vi "Periodic Tasks.vi"(8 "error in":errorcluster) -> ()   [LabVIEW 2023]
doc: "This VI runs in parallel to other tasks. It can contain as many user-defined periodic loops as you need. These can carry out PID or other sorts of timed response."
uses:
  <vilib>/Rock Robotics/WPI/DriverStation/WPI_DriverStationAllianceInfo.ctl
  <vilib>/Rock Robotics/Network Tables/NT Read String.vi
  <vilib>/Rock Robotics/Network Tables/NT Write String.vi
  GeneralPurpose/AllianceColorGlobal.vi
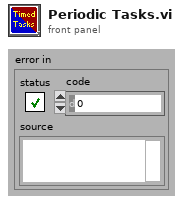
[diagram p1: front panel]
types:
  T1 = typedef "WPI_DriverStationAllianceInfo.ctl" = enum16{"Red", "Blue", "Invalid"}
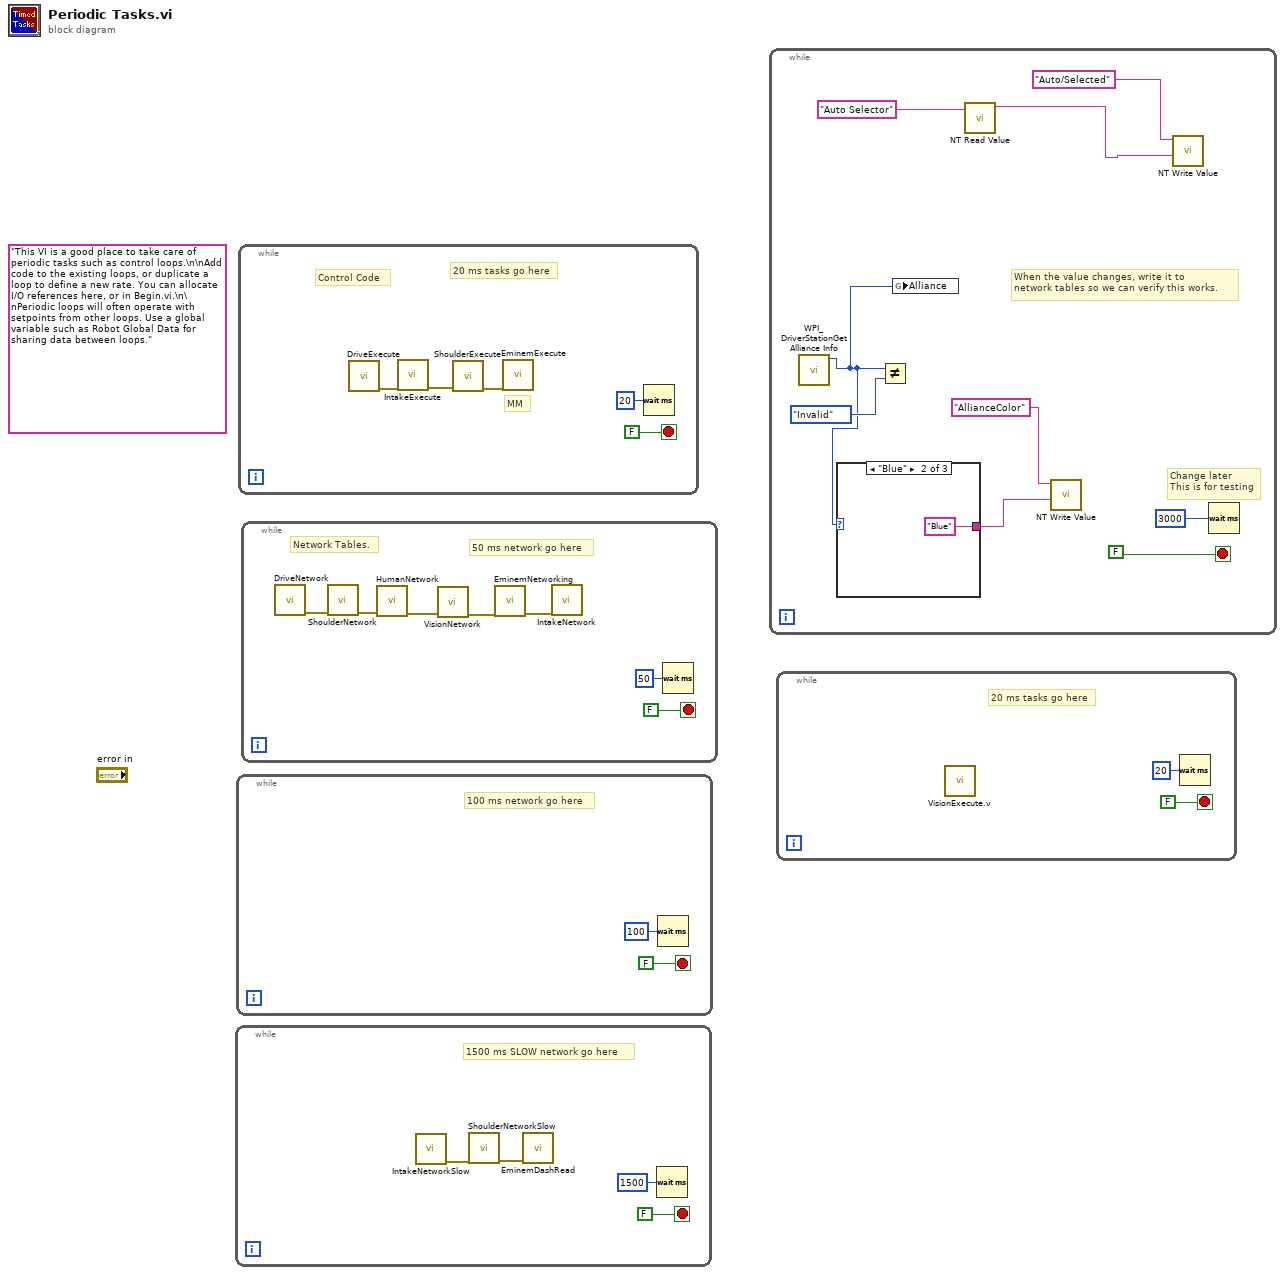
[diagram p0: block diagram]
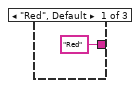
[diagram p2: hidden frame]
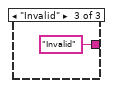
[diagram p3: hidden frame]
diagram:
  (unwired) "This VI is a good place to take care of periodic tasks such as control loops.\n\nAdd code to the existing loops, or duplicate a loop to define a new rate. You can allocate I/O references here, or in Begin.vi.\n\nPeriodic loops will often operate with setpoints from other loops. Use a global variable such as Robot Global Data for sharing data between loops."
  n1 = while {
    stop <- FALSE stop-if-true
    # "1500 ms SLOW network go here"
    n2 = call "IntakeNetworkSlow.vi"() -> ("error out"=w2:errorcluster)  [unwired: 11 in]
    n3 = call "ShoulderNetworkSlow.vi"("error in (no error)"=w2) -> ("error out"=w1:errorcluster)  [unwired: 10 in]
    n4 = call "EminemDashRead.vi"("error in (no error)"=w1) -> ()  [unwired: 10 in, 1 out]
    n5 = Wait (ms)(milliseconds to wait=u32 1500) -> ()  [unwired: 1 out]
  }
  n6 = while {
    stop <- FALSE stop-if-true
    # "100 ms network go here"
    n7 = Wait (ms)(milliseconds to wait=u32 100) -> ()  [unwired: 1 out]
  }
  n8 = while {
    stop <- FALSE stop-if-true
    # "MM"
    # "Control Code"
    # "20 ms tasks go here"
    n9 = call "DriveExecute.vi"() -> ("error out"=w9:errorcluster)  [unwired: 11 in]
    n10 = call "IntakeExecute.vi"("error in (no error)"=w9) -> ("error out"=w8:errorcluster)  [unwired: 10 in]
    n11 = call "ShoulderExecute.vi"("error in (no error)"=w8) -> ("error out"=w7:errorcluster)  [unwired: 10 in]
    n12 = call "EminemExecute.vi"("error in (no error)"=w7) -> ()  [unwired: 10 in, 1 out]
    n13 = Wait (ms)(milliseconds to wait=u32 20) -> ()  [unwired: 1 out]
  }
  n14 = while {
    stop <- FALSE stop-if-true
    # "Network Tables."
    # "50 ms network go here"
    n15 = call "DriveNetwork.vi"() -> ("error out"=w16:errorcluster)  [unwired: 11 in]
    n16 = call "ShoulderNetwork.vi"("error in (no error)"=w16) -> ("error out"=w15:errorcluster)  [unwired: 10 in]
    n17 = call "HumanNetwork.vi"("error in (no error)"=w15) -> ("error out"=w14:errorcluster)  [unwired: 10 in]
    n18 = call "VisionNetwork.vi"("error in (no error)"=w14) -> ("error out"=w13:errorcluster)  [unwired: 10 in]
    n19 = call "EminemNetworking.vi"("error in (no error)"=w13) -> ("error out"=w12:errorcluster)  [unwired: 10 in]
    n20 = call "IntakeNetwork.vi"("error in (no error)"=w12) -> ()  [unwired: 10 in, 1 out]
    n21 = Wait (ms)(milliseconds to wait=u32 50) -> ()  [unwired: 1 out]
  }
  n22 = while {
    stop <- FALSE stop-if-true
    # "When the value changes, write it to \nnetwork tables so we can verify this works."
    # "Change later\nThis is for testing"
    n23 = call <vilib>:"WPI_DriverStationGet Alliance Info.vi"() -> ("Alliance"=w24:T1)  [unwired: 6 in, 5 out]
    n24 = case shown="\"Blue\"" w24 {
      tunnel: ["Red" "Blue" "Invalid"] -> w23
      frame "Red", Default {
      }
      frame "Blue" {
      }
      frame "Invalid" {
      }
    }
    n25 = Not Equal?(x=w24, y=WPI_DriverStationAllianceInfo."Invalid") -> ()  [unwired: 1 out]
    n26 = global write "AllianceColorGlobal.vi" "Alliance"(w24) -> ()
    n27 = call-poly <vilib>:"NT Read Value.vi"("name"="Auto Selector" ("Name")) -> ("value"=w19:string)  [unwired: 8 in, 2 out]
    n28 = call-poly <vilib>:"NT Write Value.vi"("value"=w23, "name"="AllianceColor") -> ()  [unwired: 9 in, 1 out]
    n29 = call-poly <vilib>:"NT Write Value.vi"("value"=w19, "name"="Auto/Selected") -> ()  [unwired: 9 in, 1 out]
    n30 = Wait (ms)(milliseconds to wait=u32 3000) -> ()  [unwired: 1 out]
  }
  n31 = while {
    stop <- FALSE stop-if-true
    # "20 ms tasks go here"
    n32 = call "VisionExecute.v.vi"() -> ()  [unwired: 12 in]
    n33 = Wait (ms)(milliseconds to wait=u32 20) -> ()  [unwired: 1 out]
  }
